vi "2f Filter.vi"(8 "error in (no error)":errorcluster, 9 "Width":dbl=1.0, 10 "Signal":cdb[](array[numeric]), 11 "Lock-in Detector in":refnum<class "Lock-in Detector.lvclass">) -> (0 "error out":errorcluster, 2 "Signal out":cdb[](array[numeric]), 3 "Lock-in Detector out":refnum<class "Lock-in Detector.lvclass">)   [LabVIEW 2021, in "Lock-in Detector.lvclass"]
uses:
  Lock-in Detector.lvclass
  Lock-in Detector.lvclass/Lock-in Detector.ctl
  <vilib>/measure/NI_MAPro.lvlib
  <vilib>/measure/macond.llb/IIR Filter for 1 Chan (CDB).vi
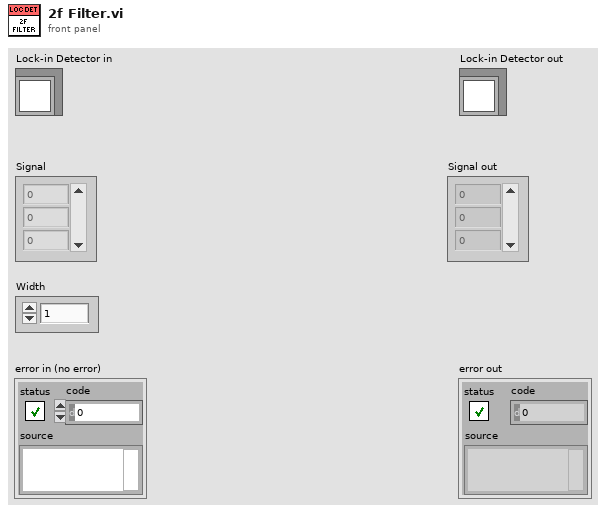
[diagram p1: front panel]
types:
  T1 = cluster{"Topology":enum16{"Off", "Butterworth", "Chebyshev", "Inverse Chebyshev", "Elliptic", "Bessel"}, "Type":enum16{"Lowpass", "Highpass", "Bandpass", "Bandstop"}, "Order":i32, "Lower Fc":dbl, "Upper Fc":dbl, "PB Ripple":dbl, "SB Attenuation":dbl}
  T2 = typedef "Lockin Parameters.ctl" = cluster{"Frequency":dbl, "Phase":dbl, "Syncronous":bool, "Points per sine wave":i32, "DDS":bool, "Frequency word":u32, "Phase word":u32, "DDS modulus":i64, "DDS clock":dbl}
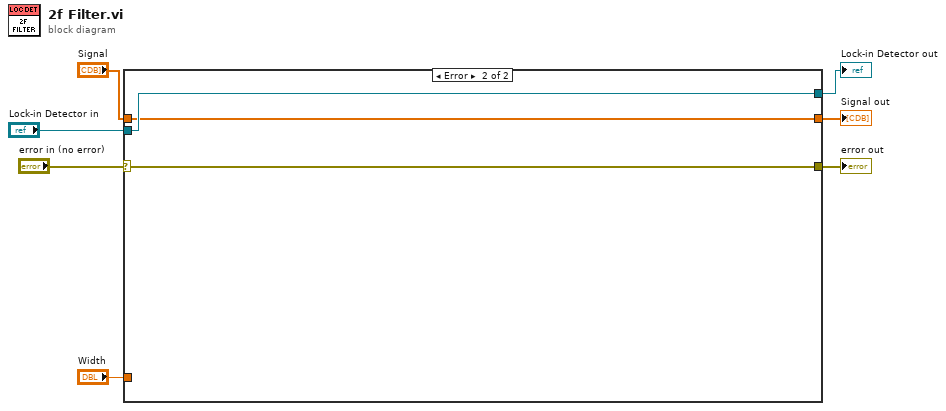
[diagram p0: block diagram]
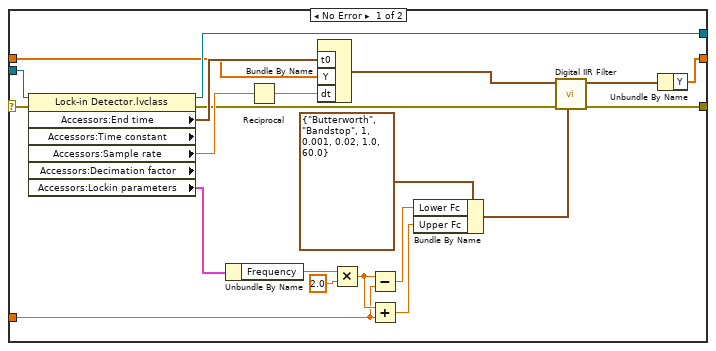
[diagram p2: hidden frame]
diagram:
  n1 = case shown="Error" "error in (no error)" {
    selector: "error in (no error)" -> [w26 w31]
    tunnel: [w10 w31] -> w6
    tunnel: [w28 w30] -> w4
    tunnel: "Lock-in Detector in" -> [w27 w30]
    tunnel: "Signal" -> [w24 w29]
    tunnel: "Width" -> [w14 _]
    tunnel: [w8 w29] -> w1
    frame No Error {
      n2 = property class="Lock-in Detector.lvclass" props=["Accessors:End time", "Accessors:Time constant", "Accessors:Sample rate", "Accessors:Decimation factor", "Accessors:Lockin parameters"](reference=w27, error in=w26) -> (reference out=w28:refnum<class "Lock-in Detector.lvclass">, error out=w11:errorcluster, "Accessors:End time"=w25:timestamp, "Accessors:Sample rate"=w23:dbl, "Accessors:Lockin parameters"=w19:T2)  [unwired: 2 out]
      n3 = Unbundle By Name(w19) -> ("Frequency"=w18:dbl)
      n4 = Reciprocal(x=w23) -> (1/x=w22:dbl)
      n5 = Bundle By Name("t0"=w25, "Y"=w24, "dt"=w22) -> (w21:waveform(cdb))  [unwired: 1 in]
      n6 = Multiply(x=w18, y=2.0) -> (x*y=w15:dbl)
      n7 = Subtract(x=w15, y=w14) -> (x-y=w16:dbl)
      n8 = Add(x=w15, y=w14) -> (x+y=w13:dbl)
      n9 = Bundle By Name(cluster=T1 {"Topology"=enum."Butterworth", "Type"=enum."Bandstop", "Order"=1, "Lower Fc"=0.001, "Upper Fc"=0.02, "PB Ripple"=1.0, "SB Attenuation"=60.0} ("IIR filter specifications"), "Lower Fc"=w16, "Upper Fc"=w13) -> (w12:T1)
      n10 = call-poly <vilib>:"Digital IIR Filter.vi"("IIR filter specifications"=w12, "error in (no error)"=w11, "signal in"=w21) -> ("error out"=w10:errorcluster, "signal out"=w9:waveform(cdb))  [unwired: 6 in, 1 out]
      n11 = Unbundle By Name(w9) -> ("Y"=w8:cdb[])
    }
    frame Error {
    }
  }
  "error out" <- w6
  "Lock-in Detector out" <- w4
  "Signal out" <- w1
